vi "Sort Data by Sort Property.vi"(7 "Connection Refnum":T1, 8 "error in (no error)":errorcluster, 10 "Sort Property Name":string, 11 "Table":T2[](array[typedef])) -> (0 "error out":errorcluster, 2 "Numeric":i32, 3 "Table 2":T2[](array[typedef]))   [LabVIEW 2011]
uses:
  CGI SimpleStat Results.ctl
  SI.LIB/ODBC/SQL Controls/Connection Refnum.ctl
  OpenG.LIB/array/array.llb/Sort 1D Array (String)__ogtk.vi
  OpenG.LIB/array/array.llb/Remove Duplicates from 1D Array (String)__ogtk.vi
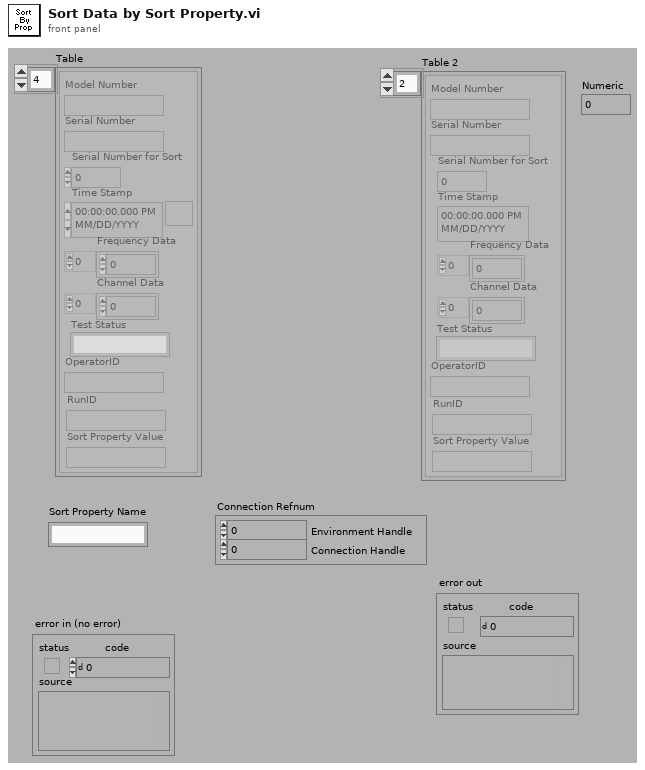
[diagram p1: front panel]
types:
  T1 = typedef "Connection Refnum.ctl" = cluster{"Environment Handle":i32, "Connection Handle":i32}
  T2 = typedef "CGI SimpleStat Results.ctl" = cluster{"Model Number":string, "Serial Number for Sort":i32, "Serial Number":string, "Time Stamp":timestamp, "Channel Data":dbl[], "Test Status":string, "OperatorID":string, "Frequency Data":dbl[], "RunID":string, "Sort Property Value":string}
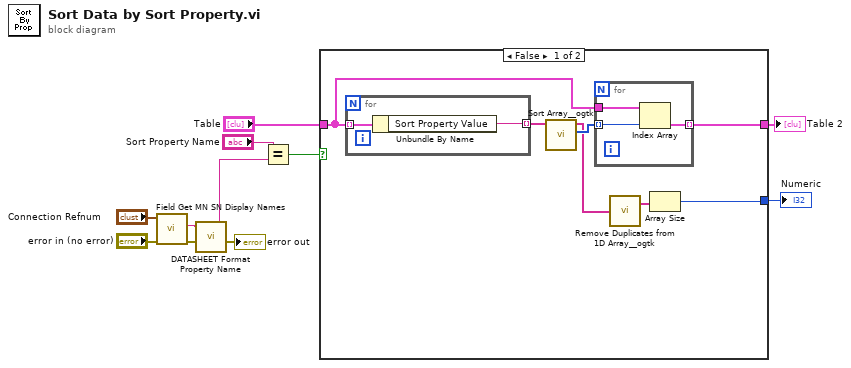
[diagram p0: block diagram]
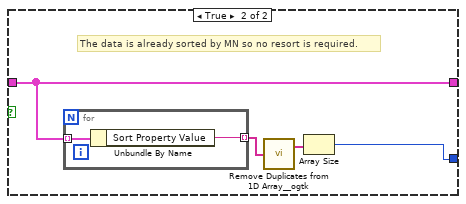
[diagram p2: hidden frame]
diagram:
  n1 = call "Field Get MN SN Display Names.vi"("error in (no error)"="error in (no error)", "Connection Refnum"="Connection Refnum") -> ("error out"=→"error out":errorcluster, "Model Number Display Name"=w6:string)  [unwired: 8 out]
  n2 = call "DATASHEET Format Property Name.vi"("String with \\r or \\n"=w6) -> ("String without \\r or \\n"=w5:string)  [unwired: 4 out]
  n3 = Equal?(x="Sort Property Name", y=w5) -> (x = y?=w7:bool)
  n4 = case shown="False" w7 {
    tunnel: "Table" -> [w16 w26]
    tunnel: [w14 w26] -> w9
    tunnel: [w11 w23] -> w2
    frame False {
      n5 = for {
        tunnel: w16 -> [w22] mode=indexing
        tunnel: [w21] -> w17 mode=indexing
        n6 = Unbundle By Name(w22) -> ("Sort Property Value"=w21:string)
      }
      n7 = call-poly "Sort Array__ogtk.vi"("Array in"=w17) -> ("Sorted Pointers"=w15:i32[], "Sorted Array out"=w13:string[])  [unwired: 1 in, 8 out]
      n8 = for {
        tunnel: w16 -> [w20]
        tunnel: w15 -> [w19] mode=indexing
        tunnel: [w18] -> w14 mode=indexing
        n9 = Index Array(array=w20, index=w19) -> (element=w18:T2)
      }
      n10 = call-poly "Remove Duplicates from 1D Array__ogtk.vi"("Input Array"=w13) -> ("Output Array"=w12:string[])  [unwired: 1 out]
      n11 = Array Size(array=w12) -> (size(s)=w11:i32)
    }
    frame True {
      # "The data is already sorted by MN so no resort is required."
      n12 = for {
        tunnel: w26 -> [w28] mode=indexing
        tunnel: [w27] -> w24 mode=indexing
        n13 = Unbundle By Name(w28) -> ("Sort Property Value"=w27:string)
      }
      n14 = call-poly "Remove Duplicates from 1D Array__ogtk.vi"("Input Array"=w24) -> ("Output Array"=w25:string[])  [unwired: 1 out]
      n15 = Array Size(array=w25) -> (size(s)=w23:i32)
    }
  }
  "Table 2" <- w9
  "Numeric" <- w2
